vi "set_config_cluster.vi"(8 "error in (no error)":errorcluster, 10 "config cluster variant":variant, 11 "TrajectoryMG100122AODFrameScan in":refnum<class "TrajectoryMH100122AODRAPS.lvclass">) -> (0 "error out":errorcluster, 3 "TrajectoryMG100122AODFrameScan out":refnum<class "TrajectoryMH100122AODRAPS.lvclass">)   [LabVIEW 2010, in "TrajectoryMH100122AODRAPS.lvclass"]
uses:
  TrajectoryMH100122AODRAPS.lvclass
  TrajectoryMH100122AODRAPS.lvclass/TrajectoryMH100122AODRAPS.ctl
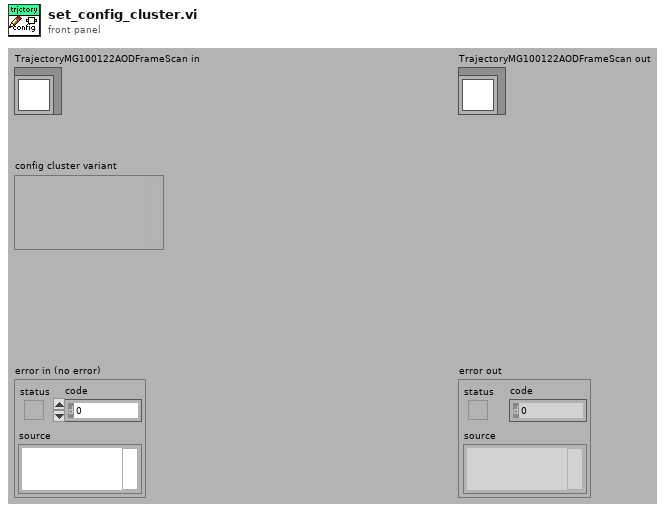
[diagram p1: front panel]
types:
  T1 = typedef "TrajectoryMH100122AODRAPS.lvclass/config_data_cluster.ctl" = cluster{"FPGA Wrapper path":cluster{"class path":string, "configuration":string, "label":string, "settings name":string}, "RAPS settings":cluster{"ROI color":u32}}
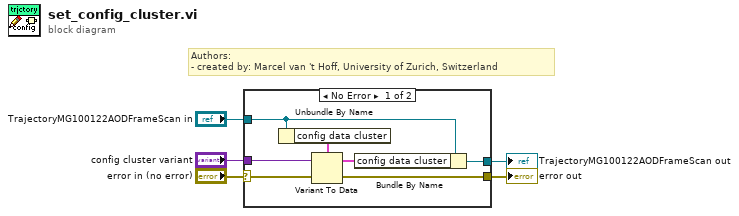
[diagram p0: block diagram]
diagram:
  # "Authors: \n- created by: Marcel van 't Hoff, University of Zurich, Switzerland"
  n1 = case shown="No Error" "error in (no error)" {
    selector: "error in (no error)" -> [w8 w14]
    tunnel: [w7 w14] -> w4
    tunnel: "TrajectoryMG100122AODFrameScan in" -> [w10 w13]
    tunnel: "config cluster variant" -> [w11 _]
    tunnel: [w6 w13] -> w1
    frame No Error {
      n2 = Unbundle By Name(w10) -> ("config data cluster"=w12:T1)
      n3 = Variant To Data(error in=w8, Variant=w11, type=w12) -> (error out=w7:errorcluster, data=w9:T1)
      n4 = Bundle By Name(cluster=w10, "config data cluster"=w9) -> (w6:refnum<class "TrajectoryMH100122AODRAPS.lvclass">)
    }
    frame Error {
    }
  }
  "error out" <- w4
  "TrajectoryMG100122AODFrameScan out" <- w1
